vi "ElevatorStateControl.vi"(9 "Elevator State":string) -> (1 "Elevator State Out":string, 2 "Target Elevator Position":dbl, 4 "Target Vacuum Pump Power":dbl)   [LabVIEW 2018]
uses:
  Inputs_DriverStation.vi
  SensorReadings.vi
  RobotStates.vi
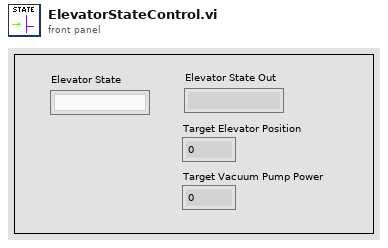
[diagram p1: front panel]
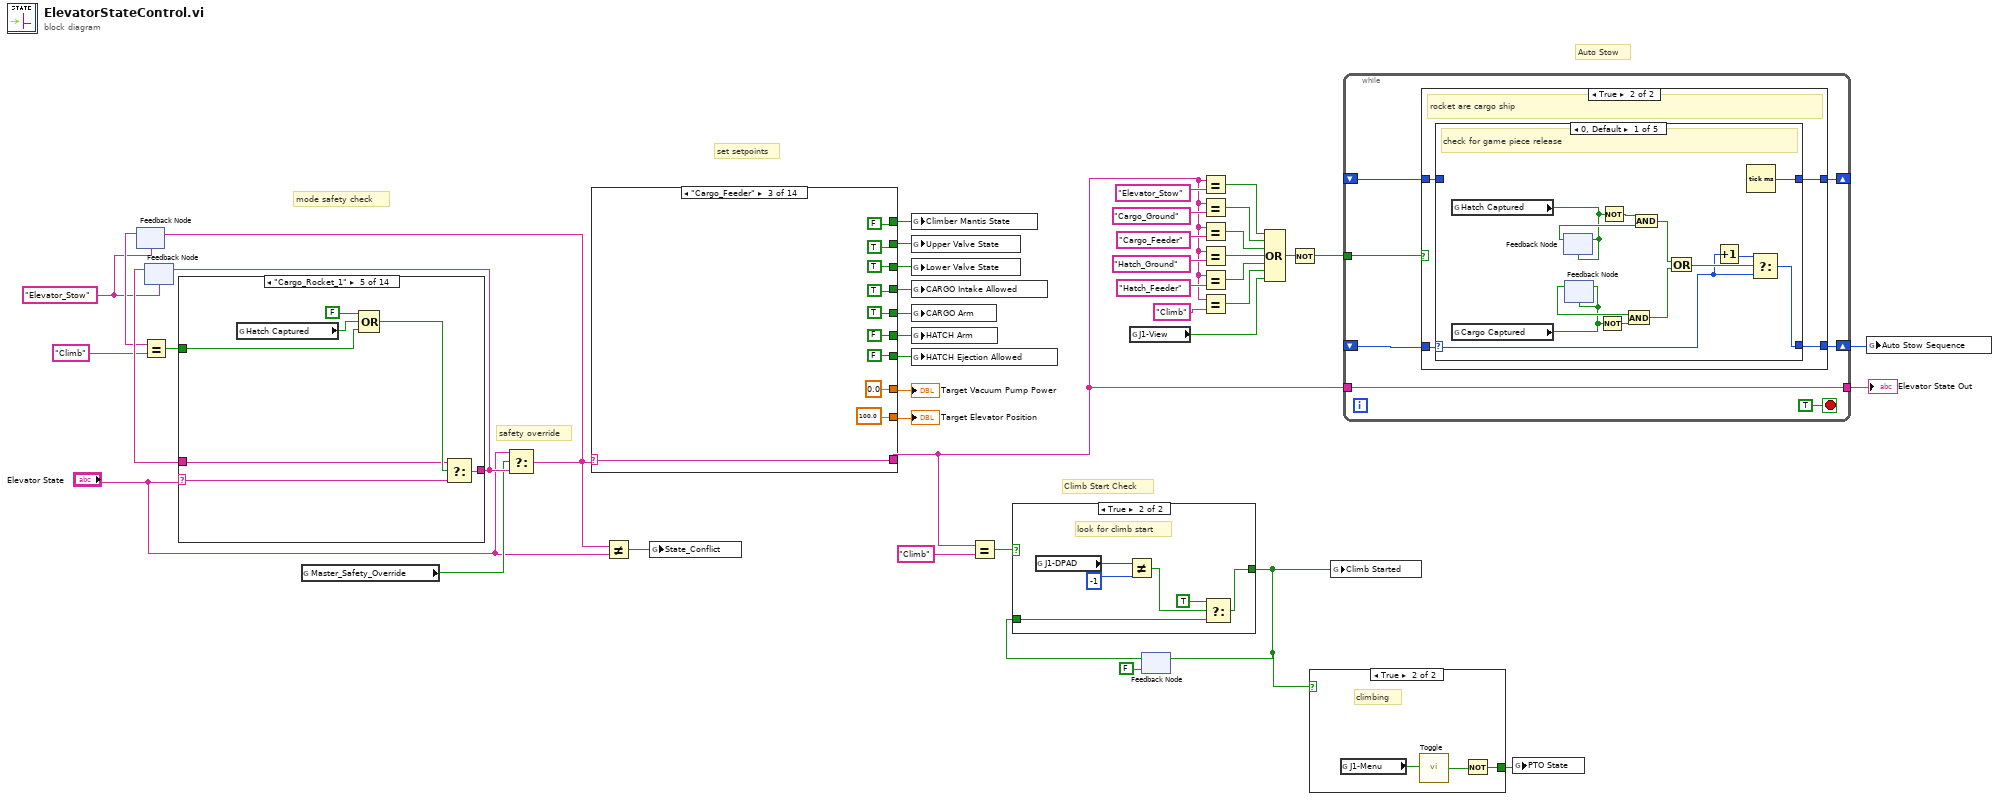
[diagram p0: block diagram]
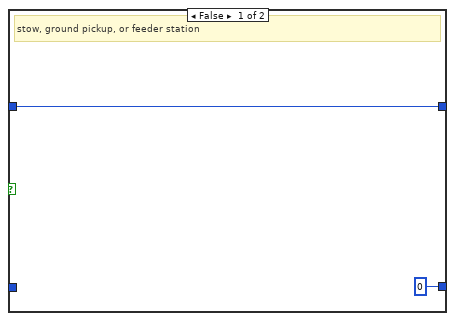
[diagram p2: hidden frame]
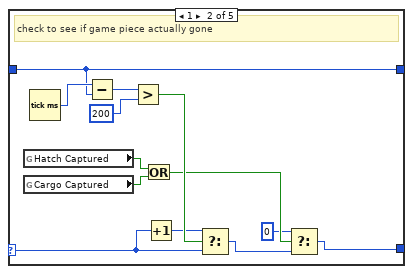
[diagram p3: hidden frame]
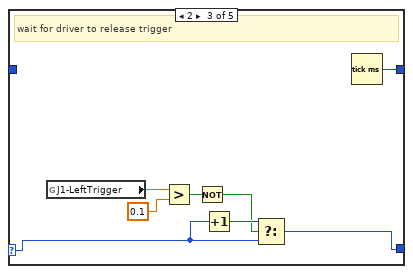
[diagram p4: hidden frame]
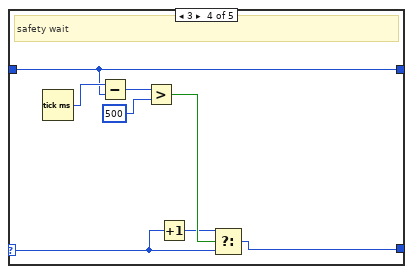
[diagram p5: hidden frame]
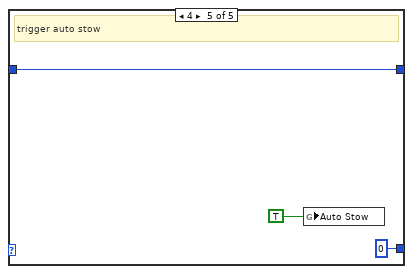
[diagram p6: hidden frame]
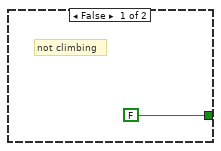
[diagram p7: hidden frame]
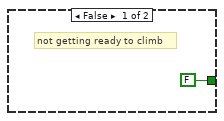
[diagram p8: hidden frame]
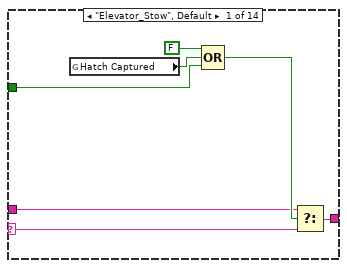
[diagram p9: hidden frame]
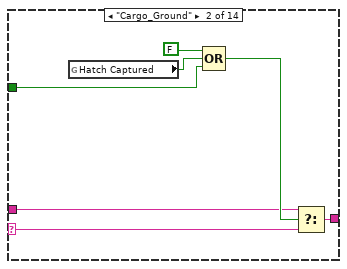
[diagram p10: hidden frame]
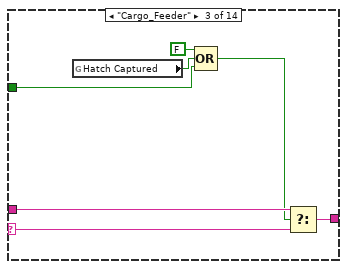
[diagram p11: hidden frame]
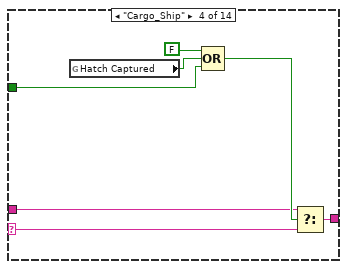
[diagram p12: hidden frame]
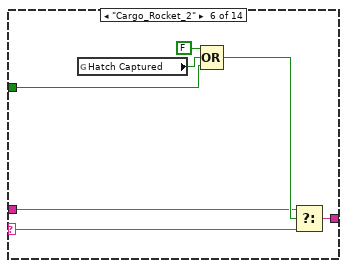
[diagram p13: hidden frame]
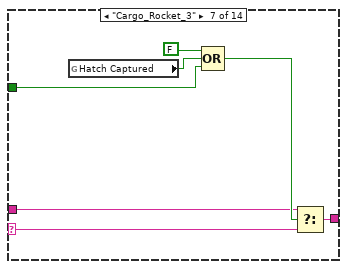
[diagram p14: hidden frame]
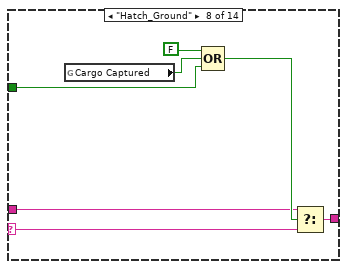
[diagram p15: hidden frame]
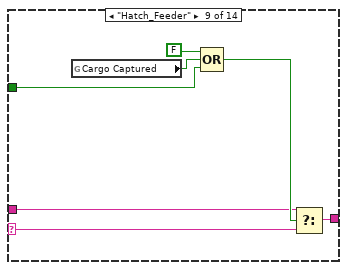
[diagram p16: hidden frame]
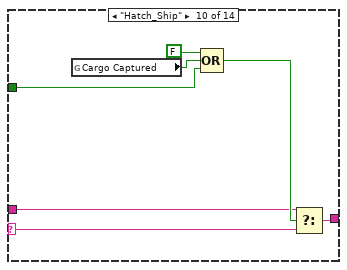
[diagram p17: hidden frame]
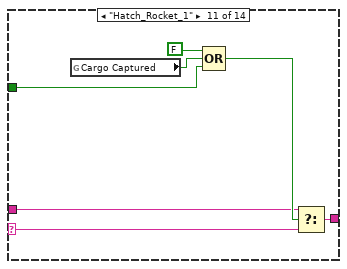
[diagram p18: hidden frame]
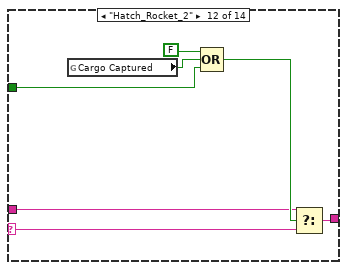
[diagram p19: hidden frame]
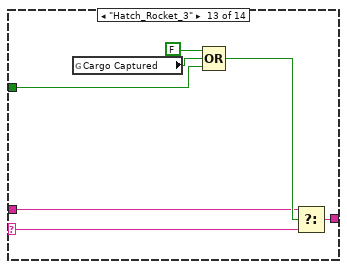
[diagram p20: hidden frame]
diagram:
  w19 = "Elevator_Stow" ("Elevator State")
  # "Auto Stow"
  # "Climb Start Check"
  # "safety override"
  # "mode safety check"
  # "set setpoints"
  n1 = feedback #1(w19) -> (w20:string)
  n2 = Equal?(x=w20, y="Climb") -> (x = y?=w28:bool)
  n3 = feedback #2(w19) -> (w30:string)
  n4 = case shown="\"Cargo_Rocket_1\"" "Elevator State" {
    selector: "Elevator State" -> [w46 w53 w64 w67 w74 w81 w89 w95 w102 w109 w116 w123 w131 w137]
    tunnel: [w48 w55 w63 w69 w76 w83 w90 w97 w104 w111 w118 w125 w132 w138] -> w37
    tunnel: w30 -> [w47 w54 w62 w68 w75 w82 w88 w96 w103 w110 w117 w124 w130 w136]
    tunnel: w28 -> [w44 w51 w58 w65 w72 w79 w86 w93 w100 w107 w114 w121 w128 _]
    frame "Elevator_Stow", Default {
      n5 = global read "SensorReadings.vi" "Hatch Captured"() -> (w45:bool)
      n6 = Compound Arithmetic op=OR(FALSE, w45, w44) -> (w49:bool)
      n7 = Select(t=w47, s=w49, f=w46) -> (s? t:f=w48:string)
    }
    frame "Cargo_Ground" {
      n8 = global read "SensorReadings.vi" "Hatch Captured"() -> (w52:bool)
      n9 = Compound Arithmetic op=OR(FALSE, w52, w51) -> (w56:bool)
      n10 = Select(t=w54, s=w56, f=w53) -> (s? t:f=w55:string)
    }
    frame "Cargo_Feeder" {
      n11 = global read "SensorReadings.vi" "Hatch Captured"() -> (w59:bool)
      n12 = Compound Arithmetic op=OR(FALSE, w59, w58) -> (w60:bool)
      n13 = Select(t=w62, s=w60, f=w64) -> (s? t:f=w63:string)
    }
    frame "Cargo_Ship" {
      n14 = global read "SensorReadings.vi" "Hatch Captured"() -> (w66:bool)
      n15 = Compound Arithmetic op=OR(FALSE, w66, w65) -> (w70:bool)
      n16 = Select(t=w68, s=w70, f=w67) -> (s? t:f=w69:string)
    }
    frame "Cargo_Rocket_1" {
      n17 = global read "SensorReadings.vi" "Hatch Captured"() -> (w73:bool)
      n18 = Compound Arithmetic op=OR(FALSE, w73, w72) -> (w77:bool)
      n19 = Select(t=w75, s=w77, f=w74) -> (s? t:f=w76:string)
    }
    frame "Cargo_Rocket_2" {
      n20 = global read "SensorReadings.vi" "Hatch Captured"() -> (w80:bool)
      n21 = Compound Arithmetic op=OR(FALSE, w80, w79) -> (w84:bool)
      n22 = Select(t=w82, s=w84, f=w81) -> (s? t:f=w83:string)
    }
    frame "Cargo_Rocket_3" {
      n23 = global read "SensorReadings.vi" "Hatch Captured"() -> (w87:bool)
      n24 = Compound Arithmetic op=OR(FALSE, w87, w86) -> (w91:bool)
      n25 = Select(t=w88, s=w91, f=w89) -> (s? t:f=w90:string)
    }
    frame "Hatch_Ground" {
      n26 = global read "SensorReadings.vi" "Cargo Captured"() -> (w94:bool)
      n27 = Compound Arithmetic op=OR(FALSE, w94, w93) -> (w98:bool)
      n28 = Select(t=w96, s=w98, f=w95) -> (s? t:f=w97:string)
    }
    frame "Hatch_Feeder" {
      n29 = global read "SensorReadings.vi" "Cargo Captured"() -> (w101:bool)
      n30 = Compound Arithmetic op=OR(FALSE, w101, w100) -> (w105:bool)
      n31 = Select(t=w103, s=w105, f=w102) -> (s? t:f=w104:string)
    }
    frame "Hatch_Ship" {
      n32 = global read "SensorReadings.vi" "Cargo Captured"() -> (w108:bool)
      n33 = Compound Arithmetic op=OR(FALSE, w108, w107) -> (w112:bool)
      n34 = Select(t=w110, s=w112, f=w109) -> (s? t:f=w111:string)
    }
    frame "Hatch_Rocket_1" {
      n35 = global read "SensorReadings.vi" "Cargo Captured"() -> (w115:bool)
      n36 = Compound Arithmetic op=OR(FALSE, w115, w114) -> (w119:bool)
      n37 = Select(t=w117, s=w119, f=w116) -> (s? t:f=w118:string)
    }
    frame "Hatch_Rocket_2" {
      n38 = global read "SensorReadings.vi" "Cargo Captured"() -> (w122:bool)
      n39 = Compound Arithmetic op=OR(FALSE, w122, w121) -> (w126:bool)
      n40 = Select(t=w124, s=w126, f=w123) -> (s? t:f=w125:string)
    }
    frame "Hatch_Rocket_3" {
      n41 = global read "SensorReadings.vi" "Cargo Captured"() -> (w129:bool)
      n42 = Compound Arithmetic op=OR(FALSE, w129, w128) -> (w133:bool)
      n43 = Select(t=w130, s=w133, f=w131) -> (s? t:f=w132:string)
    }
    frame "Climb" {
      n44 = global read "SensorReadings.vi" "Hatch Captured"() -> (w135:bool)
      n45 = global read "SensorReadings.vi" "Cargo Captured"() -> (w139:bool)
      n46 = Compound Arithmetic op=OR(FALSE, w139, w135) -> (w140:bool)
      n47 = Select(t=w136, s=w140, f=w137) -> (s? t:f=w138:string)
    }
  }
  n48 = feedback-in #2(w37) -> ()
  n49 = global read "Inputs_DriverStation.vi" "Master_Safety_Override"() -> (w36:bool)
  n50 = Select(t="Elevator State", s=w36, f=w37) -> (s? t:f=w21:string)
  n51 = feedback-in #1(w21) -> ()
  n52 = case shown="\"Cargo_Feeder\"" w21 {
    selector: w21 -> [w150 w160 w170 w180 w190 w200 w210 w219 w229 w239 w249 w259 w269 w284]
    tunnel: [FALSE TRUE TRUE TRUE TRUE TRUE TRUE FALSE FALSE FALSE FALSE FALSE FALSE FALSE] -> w43
    tunnel: [w150 w160 w170 w180 w190 w200 w210 w219 w229 w239 w249 w259 w269 w284] -> w2
    tunnel: [FALSE FALSE TRUE TRUE TRUE TRUE TRUE FALSE FALSE FALSE FALSE FALSE FALSE FALSE] -> w42
    tunnel: [w148 0.0 100.0 100.0 200.0 300.0 400.0 0.0 100.0 0.0 200.0 300.0 400.0 w275] -> w41
    tunnel: [FALSE FALSE FALSE FALSE FALSE FALSE FALSE TRUE TRUE TRUE TRUE TRUE TRUE FALSE] -> w40
    tunnel: [0.0 0.0 0.0 0.0 0.0 0.0 0.0 w215 w225 w235 w245 w255 w265 0.0 ("Vacuum_Pump")] -> w38
    tunnel: [FALSE FALSE FALSE FALSE FALSE FALSE FALSE TRUE TRUE FALSE TRUE TRUE TRUE FALSE] -> w39
    tunnel: [TRUE TRUE TRUE TRUE TRUE TRUE TRUE TRUE FALSE FALSE FALSE FALSE FALSE TRUE] -> w35
    tunnel: [TRUE TRUE TRUE TRUE TRUE TRUE TRUE FALSE TRUE TRUE TRUE TRUE TRUE TRUE] -> w34
    tunnel: [FALSE FALSE FALSE FALSE FALSE FALSE FALSE FALSE FALSE FALSE FALSE FALSE FALSE TRUE] -> w31
    frame "Elevator_Stow", Default {
      w148 = -5.0  # negative to ensure reset
    }
    frame "Cargo_Ground" {
    }
    frame "Cargo_Feeder" {
    }
    frame "Cargo_Ship" {
    }
    frame "Cargo_Rocket_1" {
    }
    frame "Cargo_Rocket_2" {
    }
    frame "Cargo_Rocket_3" {
    }
    frame "Hatch_Ground" {
      n53 = global read "Inputs_DriverStation.vi" "Vacuum_Pump"() -> (w215:dbl)
    }
    frame "Hatch_Feeder" {
      n54 = global read "Inputs_DriverStation.vi" "Vacuum_Pump"() -> (w225:dbl)
    }
    frame "Hatch_Ship" {
      n55 = global read "Inputs_DriverStation.vi" "Vacuum_Pump"() -> (w235:dbl)
    }
    frame "Hatch_Rocket_1" {
      n56 = global read "Inputs_DriverStation.vi" "Vacuum_Pump"() -> (w245:dbl)
    }
    frame "Hatch_Rocket_2" {
      n57 = global read "Inputs_DriverStation.vi" "Vacuum_Pump"() -> (w255:dbl)
    }
    frame "Hatch_Rocket_3" {
      n58 = global read "Inputs_DriverStation.vi" "Vacuum_Pump"() -> (w265:dbl)
    }
    frame "Climb" {
      w273 = 142.0  # Level 2
      w274 = 242.0  # Level 3
      n59 = global read "Inputs_DriverStation.vi" "Climb_Level"() -> (w272:bool)
      n60 = Select(t=w274, s=w272, f=w273) -> (s? t:f=w275:dbl)
    }
  }
  "Target Elevator Position" <- w41
  "Target Vacuum Pump Power" <- w38
  n61 = Not Equal?(x=w21, y="Elevator State") -> (x != y?=w32:bool)
  n62 = global write "RobotStates.vi" "State_Conflict"(w32) -> ()
  n63 = global write "RobotStates.vi" "Climber Mantis State"(w31) -> ()
  n64 = global write "RobotStates.vi" "Upper Valve State"(w35) -> ()
  n65 = global write "RobotStates.vi" "Lower Valve State"(w34) -> ()
  n66 = global write "RobotStates.vi" "CARGO Intake Allowed"(w43) -> ()
  n67 = global write "RobotStates.vi" "CARGO Arm"(w42) -> ()
  n68 = global write "RobotStates.vi" "HATCH Arm"(w40) -> ()
  n69 = global write "RobotStates.vi" "HATCH Ejection Allowed"(w39) -> ()
  n70 = Equal?(x=w2, y="Climb") -> (x = y?=w27:bool)
  n71 = global read "Inputs_DriverStation.vi" "J1-View"() -> (w4:bool)
  n72 = feedback #3(FALSE) -> (w25:bool)
  n73 = case shown="True" w27 {
    tunnel: [FALSE w289] -> w23
    tunnel: w25 -> [_ w287]
    frame False {
      # "not getting ready to climb"
    }
    frame True {
      # "look for climb start"
      n74 = global read "Inputs_DriverStation.vi" "J1-DPAD"() -> (w291:i16)
      n75 = Not Equal?(x=w291, y=i16 -1) -> (x != y?=w288:bool)
      n76 = Select(t=TRUE, s=w288, f=w287) -> (s? t:f=w289:bool)
    }
  }
  n77 = feedback-in #3(w23) -> ()
  n78 = Equal?(x=w2, y="Elevator_Stow") -> (x = y?=w18:bool)
  n79 = Equal?(x=w2, y="Cargo_Ground") -> (x = y?=w17:bool)
  n80 = Equal?(x=w2, y="Cargo_Feeder") -> (x = y?=w16:bool)
  n81 = Equal?(x=w2, y="Hatch_Ground") -> (x = y?=w15:bool)
  n82 = Equal?(x=w2, y="Hatch_Feeder") -> (x = y?=w14:bool)
  n83 = Equal?(x=w2, y="Climb") -> (x = y?=w13:bool)
  n84 = Compound Arithmetic op=OR(w18, w17, w16, w15, w14, w13, w4) -> (w10:bool)
  n85 = Not(x=w10) -> (.not. x?=w9:bool)
  n86 = case shown="True" w23 {
    tunnel: [FALSE w295] -> w22
    frame False {
      # "not climbing"
    }
    frame True {
      # "climbing"
      n87 = global read "Inputs_DriverStation.vi" "J1-Menu"() -> (w293:bool)
      n88 = call "Toggle.vi"("Trigger"=w293) -> ("New Mode"=w294:bool)
      n89 = Not(x=w294) -> (.not. x?=w295:bool)
    }
  }
  n90 = global write "RobotStates.vi" "Climb Started"(w23) -> ()
  n91 = while {
    shift-right: [w300] -> w3
    shift-left: _ -> [w301]
    tunnel: w9 -> [w299]
    shift-right: [w298] -> _
    shift-left: _ -> [w297]
    tunnel: w2 -> [w296]
    tunnel: [w296] -> w1
    stop <- TRUE stop-if-true
    n92 = case shown="True" w299 {
      tunnel: w301 -> [_ w308]
      tunnel: [0 w307] -> w300
      tunnel: [w303 w306] -> w298
      tunnel: w297 -> [w303 w305]
      frame False {
        # "stow, ground pickup, or feeder station"
      }
      frame True {
        # "rocket are cargo ship"
        n93 = case shown="0, Default" w308 {
          selector: w308 -> [w310 w330 w341 w345 _]
          tunnel: [w312 w325 w342 w344 0 ("t")] -> w307
          tunnel: [w309 w322 w335 w343 w351] -> w306
          tunnel: w305 -> [_ w322 _ w343 w351]
          frame 0, Default {
            # "check for game piece release"
            n94 = global read "SensorReadings.vi" "Hatch Captured"() -> (w315:bool)
            n95 = global read "SensorReadings.vi" "Cargo Captured"() -> (w314:bool)
            n96 = feedback-in #4(w315) -> ()
            n97 = feedback #4(w315) -> (w321:bool)
            n98 = feedback #5(w314) -> (w320:bool)
            n99 = feedback-in #5(w314) -> ()
            n100 = Not(x=w314) -> (.not. x?=w318:bool)
            n101 = Not(x=w315) -> (.not. x?=w319:bool)
            n102 = And(x=w320, y=w318) -> (x .and. y?=w316:bool)
            n103 = And(x=w319, y=w321) -> (x .and. y?=w317:bool)
            n104 = Or(x=w317, y=w316) -> (x .or. y?=w313:bool)
            n105 = Increment(x=w310) -> (x+1=w311:i32)
            n106 = Tick Count (ms)() -> (millisecond timer value=w309:u32)
            n107 = Select(t=w311, s=w313, f=w310) -> (s? t:f=w312:i32)
          }
          frame 1 {
            # "check to see if game piece actually gone"
            n108 = global read "SensorReadings.vi" "Hatch Captured"() -> (w327:bool)
            n109 = global read "SensorReadings.vi" "Cargo Captured"() -> (w328:bool)
            n110 = Tick Count (ms)() -> (millisecond timer value=w334:u32)
            n111 = Subtract(x=w334, y=w322) -> (x-y=w333:u32)
            n112 = Greater?(x=w333, y=u32 200) -> (0:w331:bool)
            n113 = Or(x=w327, y=w328) -> (x .or. y?=w324:bool)
            n114 = Increment(x=w330) -> (x+1=w329:i32)
            n115 = Select(t=w329, s=w331, f=w330) -> (s? t:f=w326:i32)
            n116 = Select(t=0, s=w324, f=w326) -> (s? t:f=w325:i32)
          }
          frame 2 {
            # "wait for driver to release trigger"
            n117 = global read "Inputs_DriverStation.vi" "J1-LeftTrigger"() -> (w339:dbl)
            n118 = Greater?(x=w339, y=0.1) -> (0:w337:bool)
            n119 = Not(x=w337) -> (.not. x?=w336:bool)
            n120 = Increment(x=w341) -> (x+1=w340:i32)
            n121 = Select(t=w340, s=w336, f=w341) -> (s? t:f=w342:i32)
            n122 = Tick Count (ms)() -> (millisecond timer value=w335:u32)
          }
          frame 3 {
            # "safety wait"
            n123 = Tick Count (ms)() -> (millisecond timer value=w350:u32)
            n124 = Subtract(x=w350, y=w343) -> (x-y=w349:u32)
            n125 = Greater?(x=w349, y=u32 500) -> (0:w347:bool)
            n126 = Increment(x=w345) -> (x+1=w346:i32)
            n127 = Select(t=w346, s=w347, f=w345) -> (s? t:f=w344:i32)
          }
          frame 4 {
            # "trigger auto stow"
            n128 = global write "RobotStates.vi" "Auto Stow"(TRUE) -> ()
          }
        }
      }
    }
  }
  "Elevator State Out" <- w1
  n129 = global write "RobotStates.vi" "PTO State"(w22) -> ()
  n130 = global write "RobotStates.vi" "Auto Stow Sequence"(w3) -> ()
